vi "Package Path.vi"(0 "Path":path) -> (4 "Package Path":path, 6 "Build Outputs":path)   [LabVIEW 2021, in "Path Functions.lvlib"]
uses:
  Path Functions.lvlib
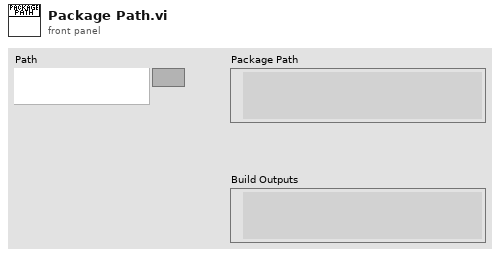
[diagram p1: front panel]
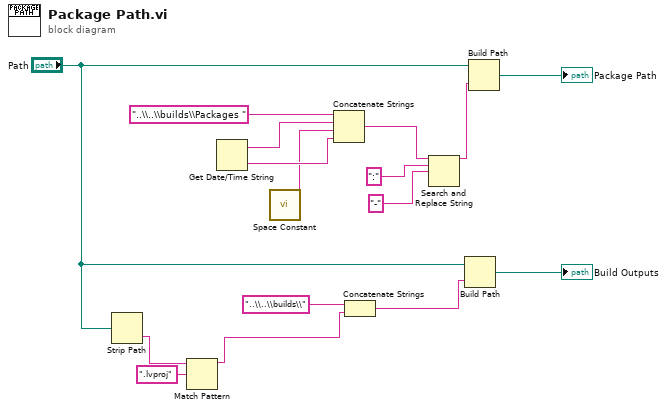
[diagram p0: block diagram]
diagram:
  n1 = Strip Path(path="Path") -> (name=w6:string)  [unwired: 1 out]
  n2 = Match Pattern(string=w6, regular expression=".lvproj") -> (before substring=w4:string)  [unwired: 1 in, 3 out]
  n3 = Get Date/Time String() -> (date string=w15:string, time string=w13:string)  [unwired: 3 in]
  n4 = call <vilib>:"Space Constant.vi"() -> ("String"=w10:string)
  n5 = Concatenate Strings("..\\..\\builds\\Packages ", w15, w10, w13) -> (w12:string)
  n6 = Concatenate Strings("..\\..\\builds\\", w4) -> (w3:string)
  n7 = Search and Replace String(input string=w12, search string=":", replace string="-" ("search string")) -> (result string=w9:string)  [unwired: 5 in, 3 out]
  n8 = Build Path(base path="Path", name or relative path=w3) -> (appended path=→"Build Outputs":path)
  n9 = Build Path(base path="Path", name or relative path=w9) -> (appended path=→"Package Path":path)
